vi "DI IRQ Initialize.vi"() -> (14 "Fatal Error Out":T11, 15 "State Out":T1)   [LabVIEW 2021, in "myRIO Register DI IRQ.xnode"]
uses:
  <vilib>/myRIO/Instrument Drivers/IRQ/IO IRQ/vis/myRIO Register DI IRQ.xnode
  <vilib>/XNodeSupport/XNodeErrorCluster.ctl
  <vilib>/myRIO/Instrument Drivers/IRQ/IO IRQ/vis/DI IRQ State.ctl
  <vilib>/myRIO/Common/Instrument Driver Framework/Utilities/typedefs/myRIOXPeripheral.ctl
  <vilib>/XNodeSupport/XNodeTerm4Array.ctl
  <vilib>/XNodeSupport/XNodeTerm4.ctl
  <vilib>/XNodeSupport/XNodeString.ctl
  <vilib>/XNodeSupport/XNodeVariant.ctl
  <vilib>/XNodeSupport/XNodeRect32.ctl
  <vilib>/XNodeSupport/XNodeInt.ctl
  <vilib>/XNodeSupport/XNodeBool.ctl
  <vilib>/XNodeSupport/XNodeTermDirection.ctl
  <vilib>/myRIO/Common/Instrument Driver Framework/myRIO v1.0/IRQ/typedefs/DI IRQ Type.ctl
  <vilib>/myRIO/Common/Instrument Driver Framework/myRIO v1.0/IRQ/typedefs/Callback VI Ref.ctl
  <vilib>/myRIO/Common/Instrument Driver Framework/Utilities/vis/myRIOXGlobal.vi
  <vilib>/XNodeSupport/NI_XNodeSupport.lvlib
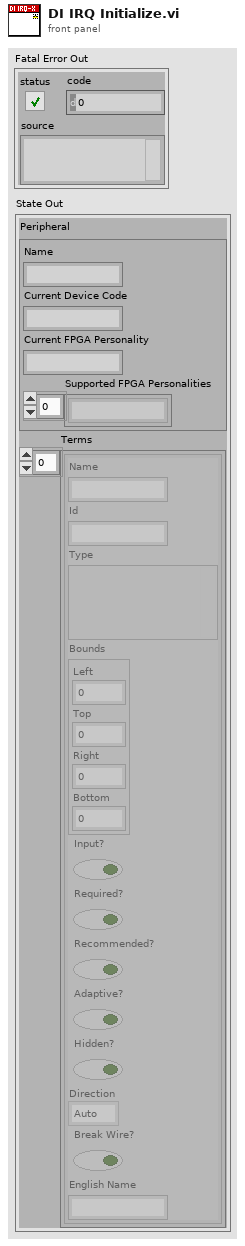
[diagram p1: front panel]
types:
  T1 = typedef "myRIO Register DI IRQ.xnode/DI IRQ State.ctl" = cluster{"Peripheral":T2, "Terms":T3}
  T2 = typedef "myRIOXPeripheral.ctl" = cluster{"Name":string, "Current Device Code":string, "Current FPGA Personality":string, "Supported FPGA Personalities":string[]}
  T3 = typedef "NI_XNodeSupport.lvlib/XNodeTerm4Array.ctl" = T4[]
  T4 = typedef "NI_XNodeSupport.lvlib/XNodeTerm4.ctl" = cluster{"Name":T5, "Id":T5, "Type":T6, "Bounds":T7, "Input?":T9, "Required?":T9, "Recommended?":T9, "Adaptive?":T9, "Hidden?":T9, "Direction":T10, "Break Wire?":T9, "English Name":T5}
  T5 = typedef "NI_XNodeSupport.lvlib/XNodeString.ctl" = string
  T6 = typedef "NI_XNodeSupport.lvlib/XNodeVariant.ctl" = variant
  T7 = typedef "NI_XNodeSupport.lvlib/XNodeRect32.ctl" = cluster{"Left":T8, "Top":T8, "Right":T8, "Bottom":T8}
  T8 = typedef "NI_XNodeSupport.lvlib/XNodeInt.ctl" = i32
  T9 = typedef "NI_XNodeSupport.lvlib/XNodeBool.ctl" = bool
  T10 = typedef "NI_XNodeSupport.lvlib/XNodeTermDirection.ctl" = enum32{"Auto", "Up", "Down", "Left", "Right", "Center"}
  T11 = typedef "NI_XNodeSupport.lvlib/XNodeErrorCluster.ctl" = errorcluster
  T12 = typedef "DI IRQ Type.ctl" = enum16{"Digital falling edge", "Digital rising edge", "Digital edge"}
  T13 = typedef "Callback VI Ref.ctl" = refnum<vi>
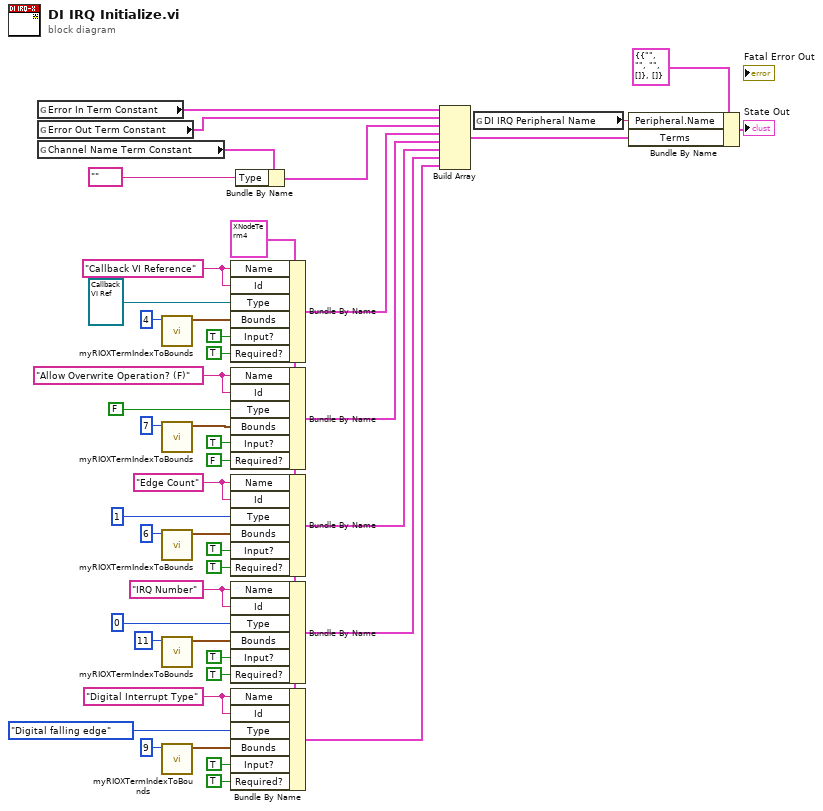
[diagram p0: block diagram]
diagram:
  w14 = T5 "Digital Interrupt Type" ("Name")
  w16 = T5 "IRQ Number" ("Name")
  w21 = T5 "Edge Count" ("Name")
  w29 = T5 "Allow Overwrite Operation? (F)" ("Name")
  w37 = T5 "Callback VI Reference" ("Name")
  w32 = T4 {"Name"="", "Id"="", "Type"=variant, "Bounds"={"Left"=0, "Top"=0, "Right"=0, "Bottom"=0}, "Input?"=FALSE, "Required?"=FALSE, "Recommended?"=FALSE, "Adaptive?"=FALSE, "Hidden?"=FALSE, "Direction"=enum."Auto", "Break Wire?"=FALSE, "English Name"=""} ("Error In Term Constant")
  n1 = global read "myRIOXGlobal.vi" "Error In Term Constant"() -> (w42:T4)
  n2 = global read "myRIOXGlobal.vi" "Error Out Term Constant"() -> (w41:T4)
  n3 = global read "myRIOXGlobal.vi" "Channel Name Term Constant"() -> (w5:T4)
  n4 = call <vilib>:"myRIOXTermIndexToBounds.vi"("Index"=4) -> ("Bounds"=w40:T7)  [unwired: 10 in]
  n5 = call <vilib>:"myRIOXTermIndexToBounds.vi"("Index"=7) -> ("Bounds"=w26:T7)  [unwired: 10 in]
  n6 = call <vilib>:"myRIOXTermIndexToBounds.vi"("Index"=6) -> ("Bounds"=w20:T7)  [unwired: 10 in]
  n7 = call <vilib>:"myRIOXTermIndexToBounds.vi"("Index"=11) -> ("Bounds"=w17:T7)  [unwired: 10 in]
  n8 = call <vilib>:"myRIOXTermIndexToBounds.vi"("Index"=9) -> ("Bounds"=w13:T7)  [unwired: 10 in]
  n9 = Bundle By Name(cluster=w32, "Name"=w37, "Id"=w37, "Type"=T13 refnum ("Callback VI"), "Bounds"=w40, "Input?"=T9 TRUE, "Required?"=T9 TRUE) -> (w35:T4)
  n10 = Bundle By Name(cluster=w32, "Name"=w29, "Id"=w29, "Type"=FALSE ("Allow Overwrite? (F)"), "Bounds"=w26, "Input?"=T9 TRUE, "Required?"=T9 FALSE) -> (w34:T4)
  n11 = Bundle By Name(cluster=w32, "Name"=w21, "Id"=w21, "Type"=u32 1 ("Edge Count"), "Bounds"=w20, "Input?"=T9 TRUE, "Required?"=T9 TRUE) -> (w33:T4)
  n12 = Bundle By Name(cluster=w32, "Name"=w16, "Id"=w16, "Type"=u8 0 ("IRQ Number"), "Bounds"=w17, "Input?"=T9 TRUE, "Required?"=T9 TRUE) -> (w31:T4)
  n13 = Bundle By Name(cluster=w32, "Name"=w14, "Id"=w14, "Type"=DI_IRQ_Type."Digital falling edge" ("DI IRQ Type"), "Bounds"=w13, "Input?"=T9 TRUE, "Required?"=T9 TRUE) -> (w30:T4)
  n14 = Bundle By Name(cluster=w5, "Type"=tag "" ("myRIO DI IRQ Channel")) -> (w4:T4)
  n15 = Build Array(w42, w41, w4, w35, w34, w33, w31, w30) -> (w3:T4[])
  n16 = global read "myRIOXGlobal.vi" "DI IRQ Peripheral Name"() -> (w43:string)
  n17 = Bundle By Name(cluster=T1 {"Peripheral"={"Name"="", "Current Device Code"="", "Current FPGA Personality"="", "Supported FPGA Personalities"=[]}, "Terms"=[]} ("State Out"), "Peripheral.Name"=w43, "Terms"=w3) -> (→"State Out":T1)
